vi "Check for Faults.vi"(8 "Error In":errorcluster caption="error in", 9 "Resistance In":dbl format="%#_6p", 10 "dmm voltage measurements":dbl[](array[numeric]), 11 "in compliance":bool[](array[boolean]) caption="smu in compliance") -> (0 "Error Out":errorcluster caption="error out", 1 "Resistance Out":dbl format="%#_6p", 2 "DMM Fault":bool, 3 "SMU Fault":bool)   [LabVIEW 2019]
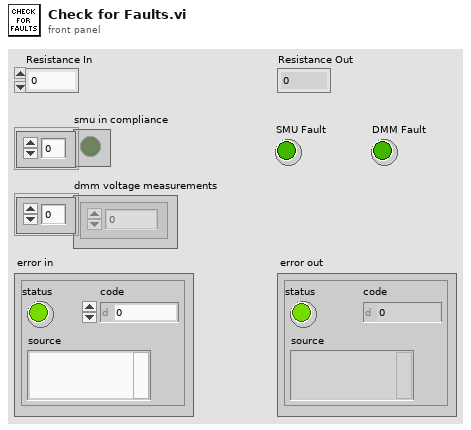
[diagram p1: front panel]
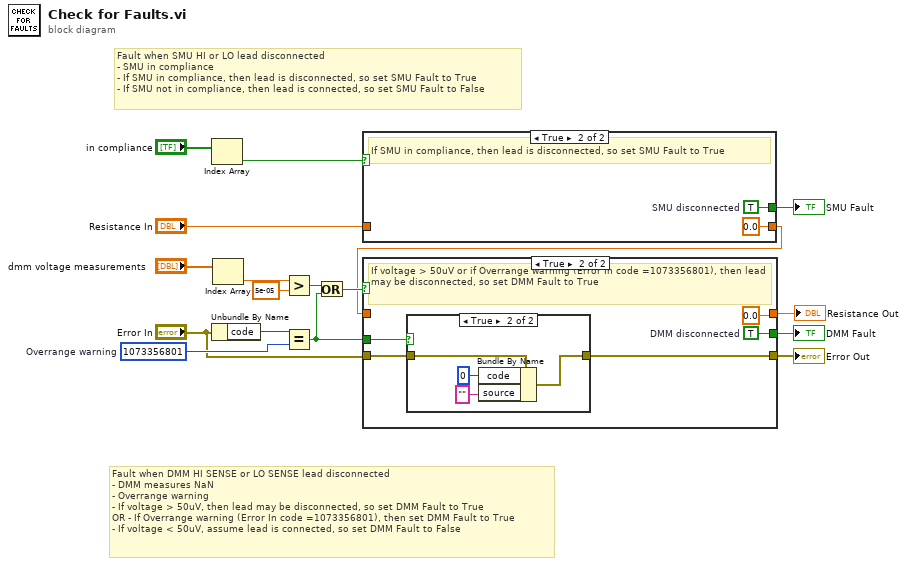
[diagram p0: block diagram]
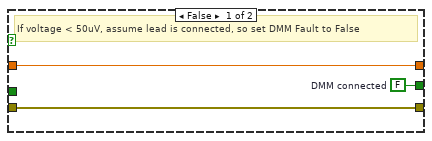
[diagram p2: hidden frame]
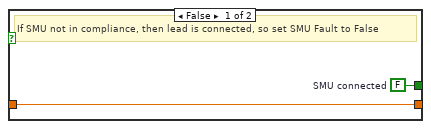
[diagram p4: hidden frame]
diagram:
  w13 = 1073356801  # Overrange warning
  # "Fault when DMM HI SENSE or LO SENSE lead disconnected\n- DMM measures NaN\n- Overrange warning\n- If voltage > 50uV, then lead may be disconnected, so set DMM Fault to True\nOR - If Overrange warning (Error In code =1073356801), then set DMM Fault to True \n- If voltage < 50uV, assume lead is connected, so set DMM Fault to False"
  # "Fault when SMU HI or LO lead disconnected\n- SMU in compliance\n- If SMU in compliance, then lead is disconnected, so set SMU Fault to True\n- If SMU not in compliance, then lead is connected, so set SMU Fault to False"
  n1 = Index Array(array="in compliance") -> (element=w7:bool)  [unwired: 1 in]
  n2 = Unbundle By Name("Error In") -> ("code"=w14:i32)
  n3 = Index Array(array="dmm voltage measurements") -> (element=w15:dbl)  [unwired: 1 in]
  n4 = Greater?(x=w15, y=5e-05) -> (0:w12:bool)
  n5 = Equal?(x=w14, y=w13) -> (x = y?=w2:bool)
  n6 = Or(x=w12, y=w2) -> (x .or. y?=w11:bool)
  n7 = case shown="True" w7 {
    tunnel: [w19 w21] -> w17
    tunnel: "Resistance In" -> [w18 _]
    tunnel: [w18 0.0 ("Resistance In")] -> w5
    frame False {
      w19 = FALSE  # SMU connected
      # "If SMU not in compliance, then lead is connected, so set SMU Fault to False"
    }
    frame True {
      w21 = TRUE  # SMU disconnected
      # "If SMU in compliance, then lead is disconnected, so set SMU Fault to True"
    }
  }
  "SMU Fault" <- w17
  n8 = case shown="True" w11 {
    tunnel: [w24 w29] -> w10
    tunnel: w5 -> [w23 _]
    tunnel: [w23 0.0 ("Resistance In")] -> w4
    tunnel: [w22 w25] -> w1
    tunnel: "Error In" -> [w22 w26]
    tunnel: w2 -> [_ w27]
    frame False {
      w24 = FALSE  # DMM connected
      # "If voltage < 50uV, assume lead is connected, so set DMM Fault to False"
    }
    frame True {
      w29 = TRUE  # DMM disconnected
      # "If voltage > 50uV or if Overrange warning (Error In code =1073356801), then lead may be disconnected, so set DMM Fault to True"
      n9 = case shown="True" w27 {
        tunnel: w26 -> [w30 w34]
        tunnel: [w30 w31] -> w25
        frame False {
        }
        frame True {
          n10 = Bundle By Name(cluster=w34, "code"=0, "source"="") -> (w31:errorcluster)
        }
      }
    }
  }
  "DMM Fault" <- w10
  "Error Out" <- w1
  "Resistance Out" <- w4
